vi "Send Msg (all).vi"(8 "error in (no error)":errorcluster, 9 "Message Data":variant, 10 "Message":string, 11 "Module Routes":refnum<user-event>[](array[refnum])) -> (0 "error out":errorcluster)   [LabVIEW 2018]
doc: "Send a message to all modules"
uses:
  Message Queue/Message Cluster.ctl
  Message Queue/Message Queue.lvlib
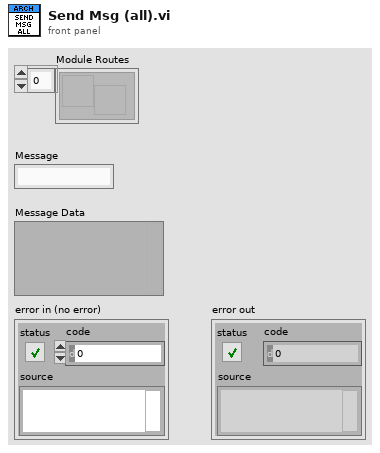
[diagram p1: front panel]
types:
  T1 = typedef "Message Queue.lvlib/Message Cluster.ctl" = cluster{"Message":string, "Message Data":variant}
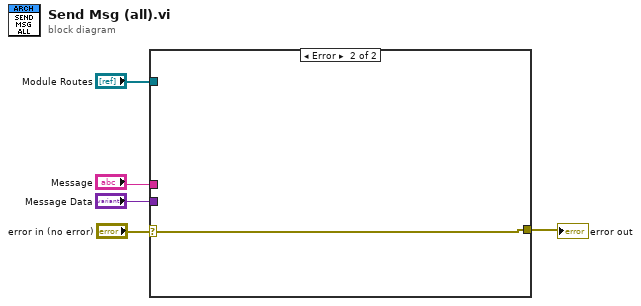
[diagram p0: block diagram]
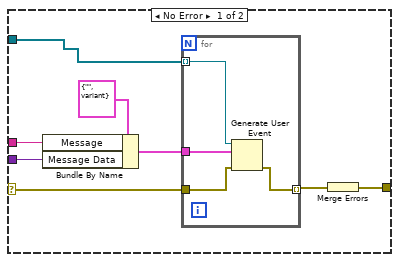
[diagram p2: hidden frame]
diagram:
  n1 = case shown="Error" "error in (no error)" {
    selector: "error in (no error)" -> [w13 w18]
    tunnel: "Module Routes" -> [w8 _]
    tunnel: "Message" -> [w10 _]
    tunnel: "Message Data" -> [w9 _]
    tunnel: [w6 w18] -> w1
    frame No Error {
      n2 = Bundle By Name(cluster=T1 {"Message"="", "Message Data"=variant} ("event data"), "Message"=w10, "Message Data"=w9) -> (w11:T1)
      n3 = for {
        tunnel: [w17] -> w7 mode=indexing
        tunnel: w13 -> [w16]
        tunnel: w11 -> [w15]
        tunnel: w8 -> [w14] mode=indexing
        n4 = Generate User Event(user event=w14, event data cluster=w15, error in=w16) -> (error out=w17:errorcluster)  [unwired: 1 in, 1 out]
      }
      n5 = Merge Errors(w7) -> (w6:errorcluster)
    }
    frame Error {
    }
  }
  "error out" <- w1
